vi "getTopicID.vi"(8 "error in (no error)":errorcluster, 10 "topic":string, 11 "ActiveMQBroker in":refnum<class "ActiveMQBroker.lvclass">) -> (0 "error out":errorcluster, 2 "topicID":u32, 3 "ActiveMQBroker out":refnum<class "ActiveMQBroker.lvclass">)   [LabVIEW 2012, in "ActiveMQBroker.lvclass"]
uses:
  <userlib>/Common/Communication/ActiveMQ/ActiveMQBroker/ActiveMQBroker.lvclass
  <userlib>/Common/Communication/ActiveMQ/ActiveMQBroker/ActiveMQBroker.lvclass/ActiveMQBroker.ctl
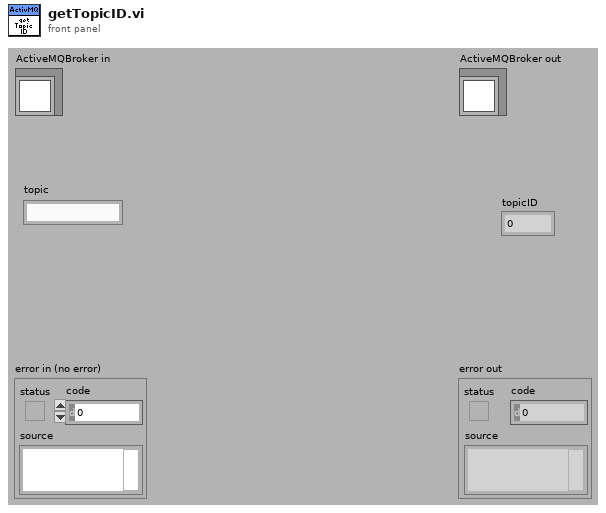
[diagram p1: front panel]
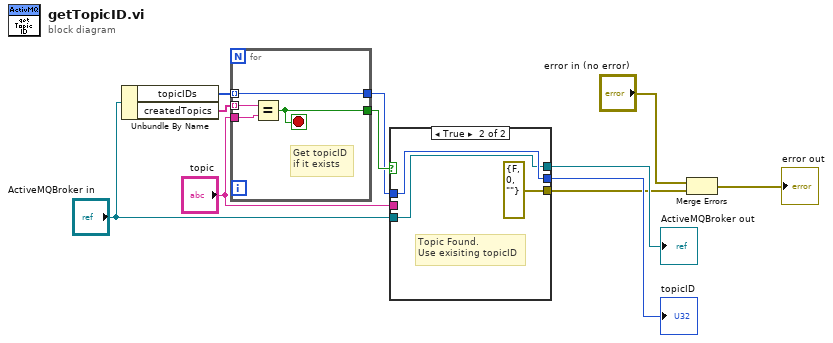
[diagram p0: block diagram]
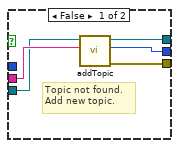
[diagram p2: hidden frame]
diagram:
  n1 = Unbundle By Name("ActiveMQBroker in") -> ("topicIDs"=w11:u32[], "createdTopics"=w10:string[])
  n2 = for {
    tunnel: w11 -> [w12] mode=indexing
    tunnel: w10 -> [w15] mode=indexing
    tunnel: "topic" -> [w14]
    tunnel: [w13] -> w9
    tunnel: [w12] -> w8
    stop <- w13 stop-if-true
    # "Get topicID\nif it exists"
    n3 = Equal?(x=w15, y=w14) -> (x = y?=w13:bool)
  }
  n4 = case shown="True" w9 {
    tunnel: w8 -> [_ w23]
    tunnel: [w17 w23] -> w7
    tunnel: "ActiveMQBroker in" -> [w19 w22]
    tunnel: "topic" -> [w20 _]
    tunnel: [w18 w22] -> w4
    tunnel: [w16 errorcluster {"status"=FALSE, "code"=0, "source"=""} ("error out")] -> w3
    frame False {
      # "Topic not found.\nAdd new topic."
      n5 = call <userlib>:"addTopic.vi"("topic"=w20, "ActiveMQBroker in"=w19) -> ("error out"=w16:errorcluster, "topicID"=w17:u32, "ActiveMQBroker out"=w18:refnum<class "ActiveMQBroker.lvclass">)  [unwired: 7 in]
    }
    frame True {
      # "Topic Found.\nUse exisiting topicID"
    }
  }
  "ActiveMQBroker out" <- w4
  "topicID" <- w7
  n6 = Merge Errors("error in (no error)", w3) -> (→"error out":errorcluster)
